vi "CMD_PDU.vi"(8 "errin":errorcluster, 11 "State?":i32 format="%.0x") -> (0 "errout":errorcluster)   [LabVIEW 2020]
uses:
  Program Files (x86)/National Instruments/LabVIEW 2020/vi.lib/Sylvain.lib/user.lib/PCAN Basic/Controls/BaudrateEenum.ctl
  <userlib>/PCAN Basic/Controls/Channel.ctl
  7e374918-bec0-49fa-a0fa-625d82639af7.vi
  <userlib>/Alex_Peak_lib/PEAK_lib_ALEX.lvlib
  <userlib>/PCAN Basic/PCANBasic.lvlib
panel:
  in  "Arrêter":bool
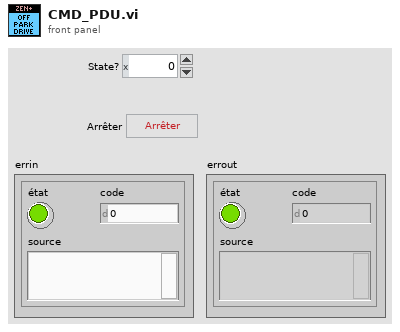
[diagram p1: front panel]
types:
  T1 = typedef "PCANBasic.lvlib/Channel.ctl" = enum16{"PCAN_NONEBUS", "not used1", "not used2", "not used3", "not used4", "not used5", "not used6", "not used7", "not used8", "not used9", "not used10", "not used11", "not used12", "not used13", "not used14", "not used15", "not used16", "not used17", "not used18", "not used19", "not used20", "not used21", "not used22", "not used23", "not used24", "not used25", "not used26", "not used27", "not used28", "not used29", "not used30", "not used31", "not used32", "PCAN_ISABUS1", "PCAN_ISABUS2", "PCAN_ISABUS3", "PCAN_ISABUS4", "PCAN_ISABUS5", "PCAN_ISABUS6", "PCAN_ISABUS7", "PCAN_ISABUS8", "not used41", "not used42", "not used43", "not used44", "not used45", "not used46", "not used47", "not used48", "PCAN_DNGBUS1", "not used50", "not used51", "not used52", "not used53", "not used54", "not used55", "not used56", "not used57", "not used58", "not used59", "not used60", "not used61", "not used62", "not used63", "not used64", "PCAN_PCIBUS1", "PCAN_PCIBUS2", "PCAN_PCIBUS3", "PCAN_PCIBUS4", "PCAN_PCIBUS5", "PCAN_PCIBUS6", "PCAN_PCIBUS7", "PCAN_PCIBUS8", "not used73", "not used74", "not used75", "not used76", "not used77", "not used78", "not used79", "not used80", "PCAN_USBBUS1", "PCAN_USBBUS2", "PCAN_USBBUS3", "PCAN_USBBUS4", "PCAN_USBBUS5", "PCAN_USBBUS6", "PCAN_USBBUS7", "PCAN_USBBUS8", "Not used89", "Not used90", "Not used91", "Not used92", "Not used93", "Not used94", "Not used95", "Not used96", "PCAN_PCCBUS1", "PCAN_PCCBUS2"}
  T2 = typedef "PCANBasic.lvlib/BaudrateEenum.ctl" = enum16{"CAN_Baud_1M", "CAN_Baud_800K", "CAN_BAUD_500K", "CAN_BAUD_250K", "CAN_BAUD_125K", "CAN_BAUD_100K", "CAN_BAUD_95K", "CAN_BAUD_83K", "CAN_BAUD_50K", "CAN_BAUD_47K", "CAN_BAUD_33K", "CAN_BAUD_20K", "CAN_BAUD_10K", "CAN_BAUD_5K", "User Baudrate"}
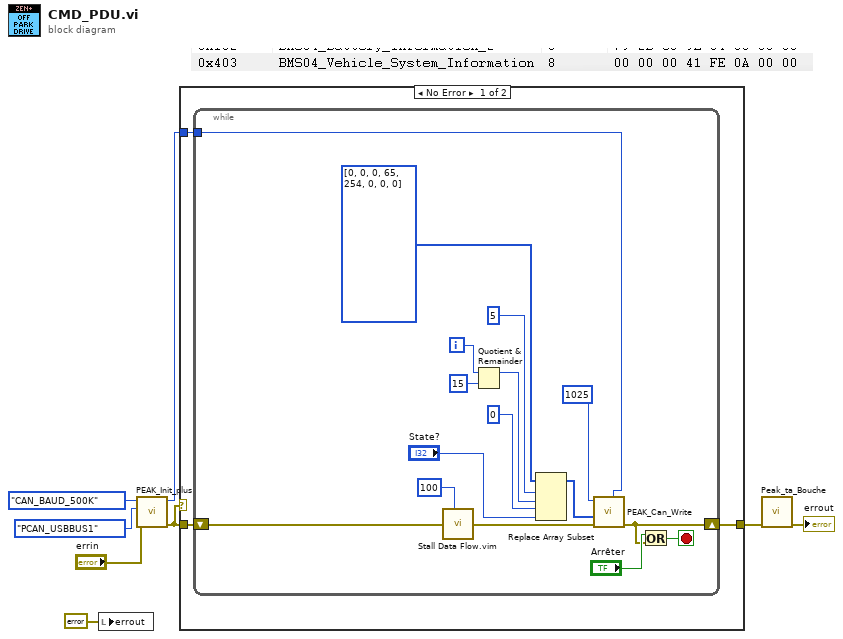
[diagram p0: block diagram]
diagram:
  n1 = local write "errout"(errorcluster {"status"=FALSE, "code"=0, "source"=""} ("errin")) -> ()
  n2 = call <userlib>:"PEAK_Init_plus.vi"("errin"="errin", "Channel"=Channel."PCAN_USBBUS1", "BTR0BTR1"=BaudrateEenum."CAN_BAUD_500K") -> ("errout"=w4:errorcluster, "Channel out"=w5:T1)  [unwired: 7 in]
  n3 = case shown="No Error" w4 {
    tunnel: w4 -> [w11 w28]
    tunnel: [w10 w28] -> w8
    tunnel: w5 -> [w9 _]
    frame No Error {
      n4 = while {
        shift-right: [w24] -> w10
        shift-left: w11 -> [w17]
        tunnel: w9 -> [w12]
        i -> [w26]
        stop <- w19 stop-if-true
        n5 = call "Stall Data Flow.vim"("value in"=w17, "milliseconds to wait"=u32 100) -> ("value out"=w16:errorcluster)  [unwired: 1 out]
        n6 = Quotient & Remainder(x=w26, y=15) -> (x-y*floor(x/y)=w21:i32)  [unwired: 1 out]
        n7 = Replace Array Subset(array=i32[] [0, 0, 0, 65, 254, 0, 0, 0], new element #1=w21, index #1=5 ("indice"), new element #2="State?", index #2=0 ("indice")) -> (w18:i32[])
        n8 = call <userlib>:"PEAK_Can_Write.vi"("CAN handle"=w12, "errin"=w16, "CAN Data"=w18, "Identifier"=u32 1025) -> ("errout"=w24:errorcluster)  [unwired: 7 in]
        n9 = Or(x="Arrêter", y=w24) -> (x .or. y?=w19:bool)
      }
    }
    frame Error {
    }
  }
  n10 = call <userlib>:"Peak_ta_Bouche.vi"("errin"=w8) -> ("sortie d'erreur"=→"errout":errorcluster)  [unwired: 8 in, 2 out]
